vi "find channel.vi"(8 "error in (no error)":errorcluster, 11 "lookup string":string) -> (0 "error out":errorcluster, 3 "channel":u16 format="%x")   [LabVIEW 2024, in "atsj peakcan basic.lvlib"]
doc: "Finds a PeakCAN <b>channel</b> that matches the specified <b>lookup string</b>."
uses:
  atsj peakcan basic.lvlib
  support/x64/PCANBasic.dll
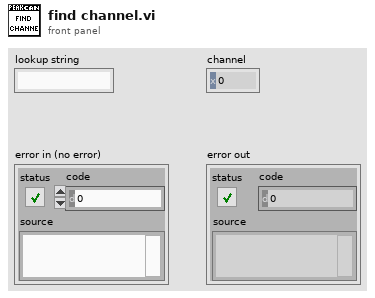
[diagram p1: front panel]
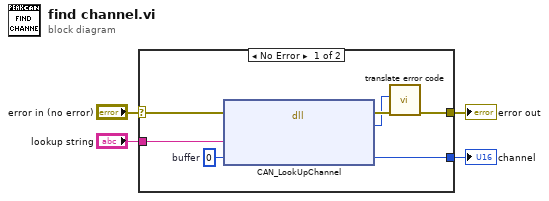
[diagram p0: block diagram]
diagram:
  n1 = case shown="No Error" "error in (no error)" {
    selector: "error in (no error)" -> [w11 w12]
    tunnel: "lookup string" -> [w8 _]
    tunnel: [w6 w12] -> w2
    tunnel: [w9 _] -> w1
    frame No Error {
      w10 = u16 0  # buffer
      n2 = dll-call lib="C:/atsj/plateau/atsj-peakcan-basic-for-labview/src/support/x64/PCANBasic.dll" fn="CAN_LookUpChannel" ("find channel")(error in=w11, "Parameters"=w8, "FoundChannel"=w10) -> (error out=w7:errorcluster, "Status"=w5:u32, "FoundChannel"=w9:u16)  [unwired: 3 in, 1 out]
      n3 = call "translate error code.vi"("error in (no error)"=w7, "error code"=w5) -> ("error out"=w6:errorcluster)  [unwired: 9 in]
    }
    frame Error {
    }
  }
  "error out" <- w2
  "channel" <- w1
